vi "PLC.Sets.Read.vi"(8 "error in":errorcluster, 11 "SettingsPath":path) -> (0 "error out":errorcluster)   [LabVIEW 2016]
uses:
  tools/Tma.lib/nlconfig.llb/fp2ini mode.ctl
  PLC.Global.vi
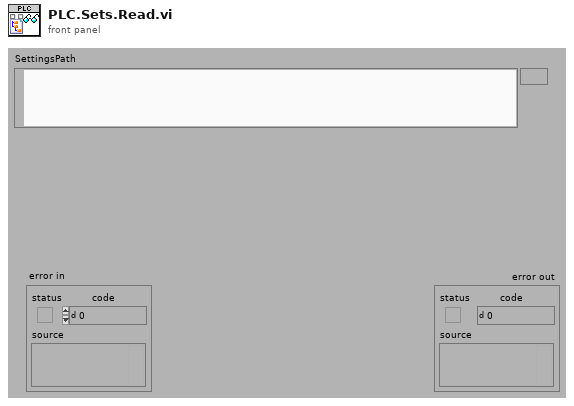
[diagram p1: front panel]
types:
  T1 = typedef "PLC.Data.Sets.ctl" = cluster{"Enable":bool, "IP":string, "Rack":i32, "Slot":i32, "LifeBitTimer_s":dbl, "DataBlockAddr_PCStatus":i32, "DataBlockAddr_PLCStatus":i32, "DataBlockAddr_PLCNewData":i32[], "DataBlockSize_PLCNewData":i32[], "DataBlockAddr_PLCChangeOver":i32[], "DataBlockSize_PLCChangeOver":i32[], "DataBlockAddr_PCChangeOver":i32[], "DataBlockAddr_PLCCheckStatus":i32[], "DataBlockSize_PLCCheckStatus":i32[], "DataBlockAddr_PCCheckStatus":i32[], "System":string}
  T2 = typedef "fp2ini mode.ctl" = enum16{"Read Controls", "Write Controls", "Write Indicators", "Read Indicators", "Write all", "Read all"}
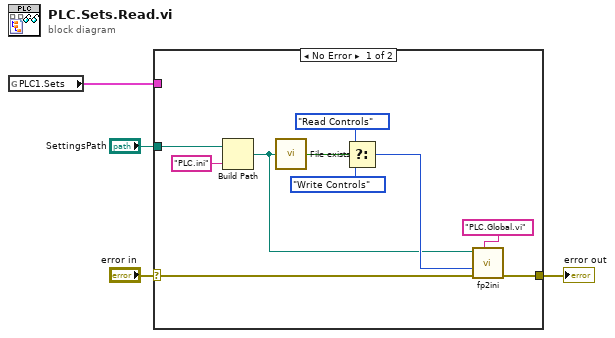
[diagram p0: block diagram]
diagram:
  n1 = global read "PLC.Global.vi" "PLC1.Sets"() -> (w1:T1)
  n2 = case shown="No Error" "error in" {
    selector: "error in" -> [w13 w15]
    tunnel: [w14 w15] -> w4
    tunnel: w1 -> [_ _]
    tunnel: "SettingsPath" -> [w6 _]
    frame No Error {
      n3 = Build Path(base path=w6, name or relative path="PLC.ini") -> (appended path=w7:path)
      n4 = call "File exists.vi"("file path"=w7) -> ("exists?"=w11:bool)  [unwired: 4 in]
      n5 = Select(t=fp2ini_mode."Read Controls" ("mode"), s=w11, f=fp2ini_mode."Write Controls" ("mode")) -> (s? t:f=w8:T2)
      n6 = call "fp2ini.vi"("vi-name (caller if empty)"="PLC.Global.vi", "error in"=w13, "mode"=w8, "ini-file path"=w7) -> ("error out"=w14:errorcluster)  [unwired: 3 in, 4 out]
    }
    frame Error {
    }
  }
  "error out" <- w4
